vi "getFAData.vi"(11 "FAILC in":refnum<class "FAILC.lvclass">) -> (2 "FAData":T1 {"Responses"."ForceAndStatus" items=["OK"=0, "IllegalFunction"=1, "IllegalDataAddress"=2, "IllegalDataValue"=3, "SlaveDeviceFailure"=4, "Acknowledge"=5, "SlaveDeviceBusy"=6, "NegativeAcknowledge"=7, "MemoryParityError"=8, "GatewayPathUnavailable"=9, "GatewayTargetDeviceFailedToRespond"=10, "WaitingForResponse"=254, "CRCError"=255]; "Responses"."SetForce" items=["OK"=0, "IllegalFunction"=1, "IllegalDataAddress"=2, "IllegalDataValue"=3, "SlaveDeviceFailure"=4, "Acknowledge"=5, "SlaveDeviceBusy"=6, "NegativeAcknowledge"=7, "MemoryParityError"=8, "GatewayPathUnavailable"=9, "GatewayTargetDeviceFailedToRespond"=10, "WaitingForResponse"=254, "CRCError"=255]; "Responses"."ReadBoosterValveGain" items=["OK"=0, "IllegalFunction"=1, "IllegalDataAddress"=2, "IllegalDataValue"=3, "SlaveDeviceFailure"=4, "Acknowledge"=5, "SlaveDeviceBusy"=6, "NegativeAcknowledge"=7, "MemoryParityError"=8, "GatewayPathUnavailable"=9, "GatewayTargetDeviceFailedToRespond"=10, "WaitingForResponse"=254, "CRCError"=255]; "Responses"."BoosterValveGain" items=["OK"=0, "IllegalFunction"=1, "IllegalDataAddress"=2, "IllegalDataValue"=3, "SlaveDeviceFailure"=4, "Acknowledge"=5, "SlaveDeviceBusy"=6, "NegativeAcknowledge"=7, "MemoryParityError"=8, "GatewayPathUnavailable"=9, "GatewayTargetDeviceFailedToRespond"=10, "WaitingForResponse"=254, "CRCError"=255]}, 3 "FAILC out":refnum<class "FAILC.lvclass">)   [LabVIEW 2016, in "RTFAILC.lvlib" / "FAILC.lvclass"]
uses:
  FAILC.lvclass
  DataTypes/FAData.ctl
  DataTypes/FAConstants.ctl
  DataTypes/FATypes.ctl
  DataTypes/FACommand.ctl
  DataTypes/FATelemetry.ctl
  DataTypes/FAResponses.ctl
  Common_RT_Modbus/DataTypes/ExceptionCodes.ctl
  DataTypes/FATimings.ctl
  DataTypes/FATimestamps.ctl
  FAILC.lvclass/FAILC.ctl
  RTFAILC.lvlib
  Common_RT_Modbus/RTModbus.lvlib
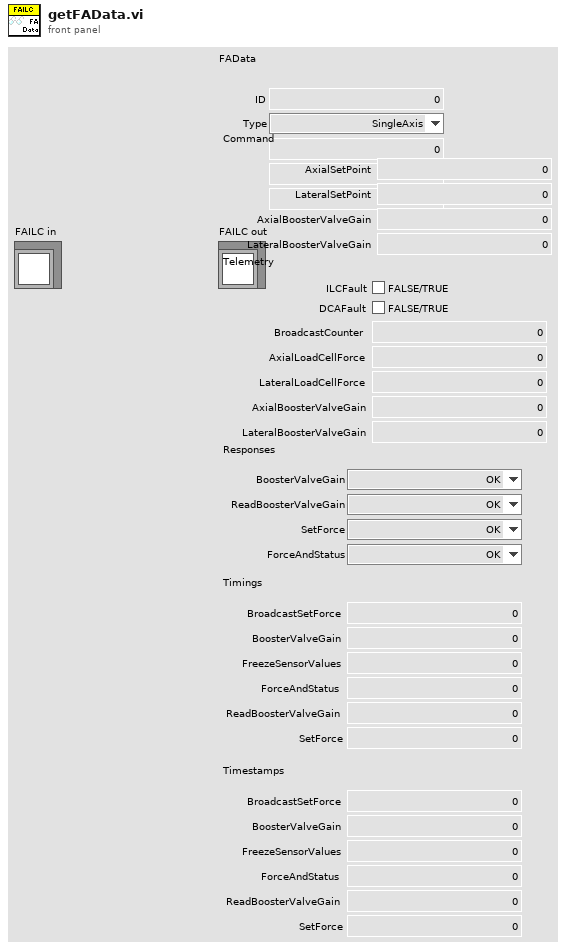
[diagram p1: front panel]
types:
  T1 = typedef "RTFAILC.lvlib/FAData.ctl" = cluster{"Constants":T2, "Command":T4, "Telemetry":T5, "Responses":T6, "Timings":T8, "Timestamps":T9}
  T2 = typedef "RTFAILC.lvlib/FAConstants.ctl" = cluster{"ID":i16, "Type":T3, "XPosition":sgl, "YPosition":sgl, "ZPosition":sgl}
  T3 = typedef "RTFAILC.lvlib/FATypes.ctl" = enum16{"SingleAxis", "DualAxis"}
  T4 = typedef "RTFAILC.lvlib/FACommand.ctl" = cluster{"AxialSetPoint":i32, "LateralSetPoint":i32, "AxialBoosterValveGain":sgl, "LateralBoosterValveGain":sgl}
  T5 = typedef "RTFAILC.lvlib/FATelemetry.ctl" = cluster{"ILCFault":bool, "DCAFault":bool, "BroadcastCounter":u8, "AxialLoadCellForce":sgl, "LateralLoadCellForce":sgl, "AxialBoosterValveGain":sgl, "LateralBoosterValveGain":sgl}
  T6 = typedef "RTFAILC.lvlib/FAResponses.ctl" = cluster{"BoosterValveGain":T7, "ReadBoosterValveGain":T7, "SetForce":T7, "ForceAndStatus":T7}
  T7 = typedef "RTModbus.lvlib/ExceptionCodes.ctl" = u16
  T8 = typedef "RTFAILC.lvlib/FATimings.ctl" = cluster{"BroadcastSetForce":u32, "BoosterValveGain":u32, "FreezeSensorValues":u32, "ForceAndStatus":u32, "ReadBoosterValveGain":u32, "SetForce":u32}
  T9 = typedef "RTFAILC.lvlib/FATimestamps.ctl" = cluster{"BroadcastSetForce":dbl, "BoosterValveGain":dbl, "FreezeSensorValues":dbl, "ForceAndStatus":dbl, "ReadBoosterValveGain":dbl, "SetForce":dbl}
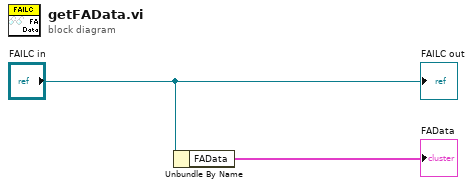
[diagram p0: block diagram]
diagram:
  n1 = Unbundle By Name("FAILC in") -> ("FAData"=→"FAData":T1)
  "FAILC out" <- "FAILC in"
